vi "Update Status Bar Init.vi"(4 "SN Value":string, 5 "MN Value":string, 6 "SN Display Name":string, 7 "MN Display Name":string, 8 "error in (no error)":errorcluster, 11 "Status Bar":refnum<vi>) -> (0 "error out":errorcluster, 3 "Status Bar Out":refnum<vi>)   [LabVIEW 2011]
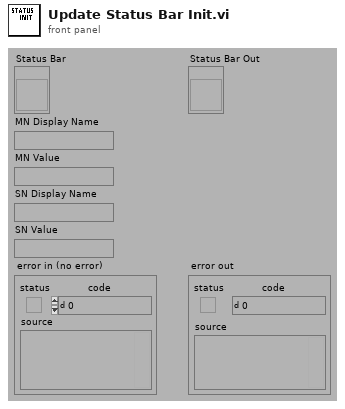
[diagram p1: front panel]
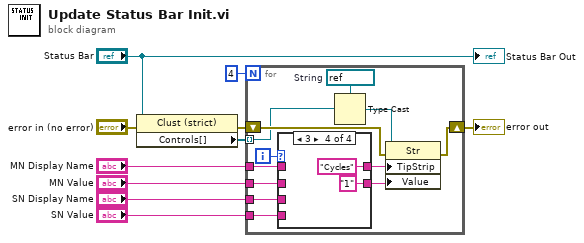
[diagram p0: block diagram]
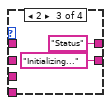
[diagram p4: hidden frame]
diagram:
  n1 = property class="Clust (strict)"(reference="Status Bar", error in="error in (no error)") -> (error out=w10:errorcluster, "Controls[]"=w2:refnum<vi>[])  [unwired: 1 out]
  n2 = for {
    N: 4 -> [_]
    shift-right: [w22] -> w8
    shift-left: w10 -> [w18]
    tunnel: "MN Display Name" -> [w15]
    tunnel: "MN Value" -> [w14]
    tunnel: "SN Display Name" -> [w13]
    tunnel: "SN Value" -> [w12]
    tunnel: w2 -> [w11] mode=indexing
    i -> [w21]
    w16 = refnum<vi> refnum  # String
    n3 = case shown="3" w21 {
      tunnel: [w24 w26 "Status" "Cycles"] -> w20
      tunnel: [w23 w25 "Initializing..." "1"] -> w19
      tunnel: w15 -> [w24 _ _ _]
      tunnel: w14 -> [w23 _ _ _]
      tunnel: w13 -> [_ w26 _ _]
      tunnel: w12 -> [_ w25 _ _]
      frame 0, Default {
      }
      frame 1 {
      }
      frame 2 {
      }
      frame 3 {
      }
    }
    n4 = Type Cast(type=w16, x=w11) -> (*(type *) &x=w17:refnum<vi>)
    n5 = property class="Str"(reference=w17, error in=w18, "TipStrip"=w20, "Value"=w19) -> (error out=w22:errorcluster)  [unwired: 1 out]
  }
  "error out" <- w8
  "Status Bar Out" <- "Status Bar"
